vi "test Factory.vi"() -> ()   [LabVIEW 2020]
uses:
  Analyze Classes/Analyze.lvlib
panel:
  out "Array 2":string[](array[string])
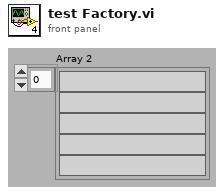
[diagram p1: front panel]
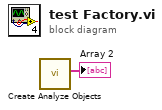
[diagram p0: block diagram]
diagram:
  n1 = call "Create Analyze Objects.vi"() -> ("Short Name"=→"Array 2":string[])  [unwired: 9 in, 2 out]
